vi "From Cluster.vi"(8 "Error In":errorcluster, 10 "Cluster Variant":variant, 11 "Tree Data Type":refnum<class "Tree Data.lvclass">) -> (0 "Error Out":errorcluster, 3 "Tree Data Out":refnum<class "Tree Data.lvclass">, 5 "Unique ID":string)   [LabVIEW 2017, in "Tree API.lvlib" / "Tree.lvclass"]
doc: "Convert the wired in cluster into a Tree representation. Only the default supported data types can be converted using this method. If your cluster contains anything more complicated than default Tree Data Types, you need to write your own low level cluster translation.\n\nThe Unique ID output will return an ID of the newly created Tree."
uses:
  Tree.lvclass
  Tree Data/Tree Data.lvclass
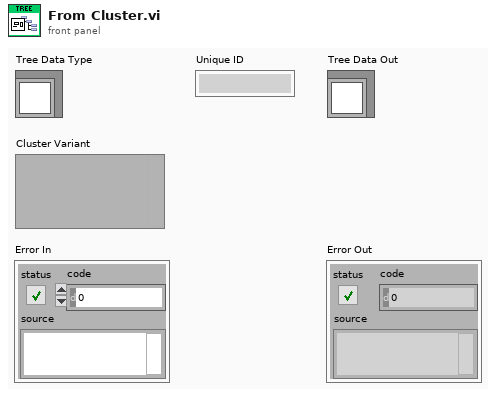
[diagram p1: front panel]
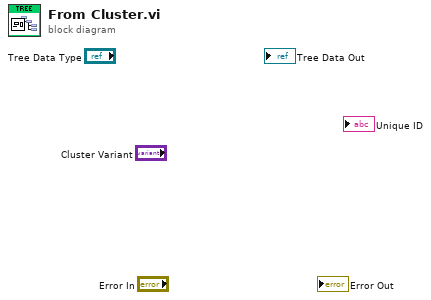
[diagram p0: block diagram]
diagram:
